vi "waitMicroseconds.vi"(8 "error in (no error)":errorcluster, 10 "Time (us)":u32, 11 "Model in":refnum<class "Model.lvclass">) -> (0 "error out":errorcluster, 3 "Model out":refnum<class "Model.lvclass">)   [LabVIEW 2016, in "Model.lvclass"]
uses:
  Model.lvclass
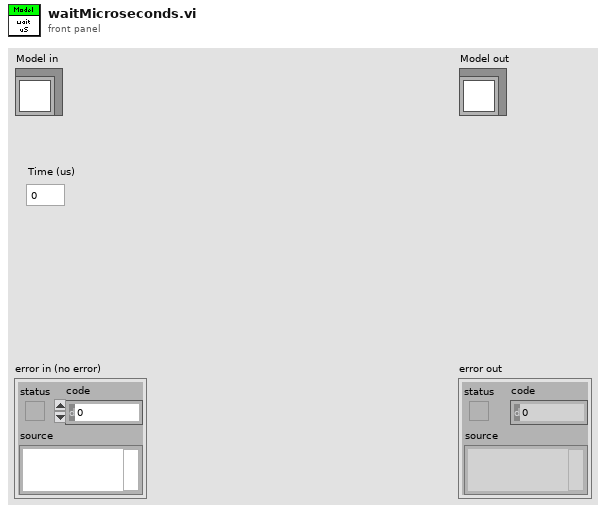
[diagram p1: front panel]
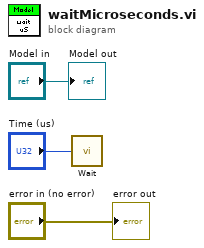
[diagram p0: block diagram]
diagram:
  n1 = call "Wait"("Count(uSec)"="Time (us)") -> ()  [unwired: 1 out]
  "error out" <- "error in (no error)"
  "Model out" <- "Model in"
